vi "_ROSDefinition.vi"() -> ()   [LabVIEW 2013]
uses:
  SubVIs/_ROSDirection.ctl
panel:
  out "Port Count":i32=9
  out "Right Gripper":T1={"Seconds"=1403708875, "NanoSec"=338000000, "ID"=65538, "enabled"=enum."TRUE", "calibrated"=enum."UNKNOWN", "ready"=enum."FALSE", "moving"=enum."TRUE", "gripping"=enum."FALSE", "missed"=enum."UNKNOWN", "error"=enum."FALSE", "reverse"=enum."FALSE", "position"=0.0, "force"=0.0, "state"="{\n  \"error_flags\" : 0,\n  \"op_mode\" : 0\n}", "command"="calibrate", "command sender"="NONA", "command sequence"=3} {"ID" format="%08x"}
  in  "Baxter Topics Old":T3(array[cluster])=[{"Topic"="/robot/head/command_head_nod", "Type"="std_msgs/Bool", "Action"=enum."Publisher"}, {"Topic"="/robot/limb/left/joint_command_mode", "Type"="baxter_msgs/JointCommandMode", "Action"=enum."Publisher"}, {"Topic"="/robot/limb/left/command_joint_angles", "Type"="baxter_msgs/JointPositions", "Action"=enum."Publisher"}, {"Topic"="/robot/limb/right/joint_command_mode", "Type"="baxter_msgs/JointCommandMode", "Action"=enum."Publisher"}, {"Topic"="/robot/limb/right/command_joint_angles", "Type"="baxter_msgs/JointPositions", "Action"=enum."Publisher"}, {"Topic"="/robot/set_super_enable", "Type"="std_msgs/Bool", "Action"=enum."Publisher"}, {"Topic"="/robot/joint_states", "Type"="sensor_msgs/JointState", "Action"=enum."Subscriber"}, {"Topic"="/robot/range/right_hand_range", "Type"="sensor_msgs/Range", "Action"=enum."Subscriber"}, {"Topic"="/robot/range/left_hand_range", "Type"="sensor_msgs/Range", "Action"=enum."Subscriber"}, {"Topic"="/cameras/left_hand_camera/image", "Type"="sensor_msgs/Image", "Action"=enum."Subscriber"}, {"Topic"="/cameras/right_hand_camera/image", "Type"="sensor_msgs/Image", "Action"=enum."Subscriber"}, {"Topic"="/cameras/head_camera/image", "Type"="sensor_msgs/Image", "Action"=enum."Subscriber"}, {"Topic"="/robot/limb/right/accessory/gripper/command_calibrate", "Type"="std_msgs/Bool", "Action"=enum."Publisher"}, {"Topic"="/robot/limb/left/accessory/gripper/command_calibrate", "Type"="std_msgs/Empty", "Action"=enum."Publisher"}, {"Topic"="/robot/limb/left/accessory/gripper/command_goto", "Type"="std_msgs/Float32", "Action"=enum."Publisher"}, {"Topic"="/robot/limb/right/accessory/gripper/command_goto", "Type"="std_msgs/Float32", "Action"=enum."Publisher"}, {"Topic"="/sdk/robot/digital_io/left_lower_cuff/state", "Type"="baxter_msgs/DigitalIOState", "Action"=enum."Subscriber"}, {"Topic"="/sdk/robot/digital_io/right_lower_cuff/state", "Type"="baxter_msgs/DigitalIOState", "Action"=enum."Subscriber"}, {"Topic"="/sdk/robot/digital_io/command", "Type"="baxter_msgs/DigitalOutputCommand", "Action"=enum."Publisher"}, {"Topic"="/sdk/robot/itb/torso_left_itb/state", "Type"="baxter_msgs/ITB", "Action"=enum."Subscriber"}, {"Topic"="/sdk/robot/itb/left_itb/state", "Type"="baxter_msgs/ITB", "Action"=enum."Subscriber"}, {"Topic"="/sdk/robot/itb/torso_right_itb/state", "Type"="baxter_msgs/ITB", "Action"=enum."Subscriber"}, {"Topic"="/sdk/robot/itb/right_itb/state", "Type"="baxter_msgs/ITB", "Action"=enum."Subscriber"}, {"Topic"="/sdk/xdisplay", "Type"="sensor_msgs/Image", "Action"=enum."Publisher"}, {"Topic"="/sdk/robot/digital_io/left_lower_button/state", "Type"="baxter_msgs/DigitalIOState", "Action"=enum."Subscriber"}, {"Topic"="/sdk/robot/digital_io/right_lower_button/state", "Type"="baxter_msgs/DigitalIOState", "Action"=enum."Subscriber"}, {"Topic"="/sdk/robot/digital_io/left_upper_button/state", "Type"="baxter_msgs/DigitalIOState", "Action"=enum."Subscriber"}, {"Topic"="/sdk/robot/digital_io/right_upper_button/state", "Type"="baxter_msgs/DigitalIOState", "Action"=enum."Subscriber"}, {"Topic"="/sdk/robot/limb/right/endpoint/state", "Type"="baxter_msgs/EndpointState", "Action"=enum."Subscriber"}, {"Topic"="/sdk/robot/limb/left/endpoint/state", "Type"="baxter_msgs/EndpointState", "Action"=enum."Subscriber"}, {"Topic"="/sdk/robot/limb/left/accessory/gripper/state", "Type"="baxter_msgs/GripperState", "Action"=enum."Subscriber"}, {"Topic"="/sdk/robot/limb/right/accessory/gripper/state", "Type"="baxter_msgs/GripperState", "Action"=enum."Subscriber"}, {"Topic"="/joint_states", "Type"="sensor_msgs/JointState", "Action"=enum."Subscriber"}, {"Topic"="/sdk/robot/limb/left/solve_ik_position", "Type"="baxter_msgs/SolvePositionIK", "Action"=enum."Service Client"}, {"Topic"="/sdk/robot/limb/right/solve_ik_position", "Type"="baxter_msgs/SolvePositionIK", "Action"=enum."Service Client"}, {"Topic"="/cameras/close", "Type"="baxter_msgs/CloseCamera", "Action"=enum."Service Client"}, {"Topic"="/cameras/open", "Type"="baxter_msgs/OpenCamera", "Action"=enum."Service Client"}, {"Topic"="/cameras/list", "Type"="baxter_msgs/ListCameras", "Action"=enum."Service Client"}, {"Topic"="/robot/sonar/head_sonar/state", "Type"="sensor_msgs/PointCloud", "Action"=enum."Subscriber"}, {"Topic"="/robot/limb/left/command_joint_velocities", "Type"="std_msgs/JointVelocities", "Action"=enum."Publisher"}, {"Topic"="/robot/limb/right/command_joint_velocities", "Type"="std_msgs/JointVelocities", "Action"=enum."Publisher"}, {"Topic"="/robot/sonar/set_lights", "Type"="std_msgs/uint16", "Action"=enum."Publisher"}, {"Topic"="/robot/sonar/set_red_level", "Type"="std_msgs/Float32", "Action"=enum."Publisher"}, {"Topic"="/robot/sonar/set_red_level", "Type"="std_msgs/Float32", "Action"=enum."Publisher"}, {"Topic"="/robot/sonar/set_green_level", "Type"="std_msgs/Float32", "Action"=enum."Publisher"}, {"Topic"="/sdk/robot/head/command_head_pan", "Type"="baxter_msgs/HeadPanCommand", "Action"=enum."Publisher"}, {"Topic"="/sdk/robot/limb/left/accessory/gripper/identity", "Type"="baxter_msgs/GripperIdentity", "Action"=enum."Subscriber"}, {"Topic"="/robot/limb/right/joint_command", "Type"="baxter_msgs/JointCommand", "Action"=enum."Publisher"}, {"Topic"="/robot/limb/left/joint_command", "Type"="baxter_msgs/JointCommand", "Action"=enum."Publisher"}]
  out "Ports":u16[](array[numeric])
  in  "FIFO Size":i32=10
  in  "Active Servers":T4(array[cluster])
  in  "Baxter Topics":T3(array[cluster])=[{"Topic"="/cameras/close", "Type"="baxter_msgs/CloseCamera", "Action"=enum."Service Client"}, {"Topic"="/cameras/head_camera/image", "Type"="sensor_msgs/Image", "Action"=enum."Subscriber"}, {"Topic"="/cameras/left_hand_camera/image", "Type"="sensor_msgs/Image", "Action"=enum."Subscriber"}, {"Topic"="/cameras/list", "Type"="baxter_msgs/ListCameras", "Action"=enum."Service Client"}, {"Topic"="/cameras/open", "Type"="baxter_msgs/OpenCamera", "Action"=enum."Service Client"}, {"Topic"="/cameras/right_hand_camera/image", "Type"="sensor_msgs/Image", "Action"=enum."Subscriber"}, {"Topic"="/joint_states", "Type"="sensor_msgs/JointState", "Action"=enum."Subscriber"}, {"Topic"="/robot/analog_io/left_hand_range/value_uint32", "Type"="std_msgs/Uint32", "Action"=enum."Subscriber"}, {"Topic"="/robot/analog_io/right_hand_range/value_uint32", "Type"="std_msgs/Uint32", "Action"=enum."Subscriber"}, {"Topic"="/robot/digital_io/right_shoulder_button/state", "Type"="baxter_core_msgs/DigitalIOState", "Action"=enum."Subscriber"}, {"Topic"="/robot/end_effector/left_gripper/command", "Type"="baxter_core_msgs/EndEffectorCommand", "Action"=enum."Publisher"}, {"Topic"="/robot/end_effector/right_gripper/command", "Type"="baxter_core_msgs/EndEffectorCommand", "Action"=enum."Publisher"}, {"Topic"="/robot/end_effector/left_gripper/state", "Type"="std_msgs/EndEffectorState", "Action"=enum."Subscriber"}, {"Topic"="/robot/end_effector/right_gripper/state", "Type"="std_msgs/EndEffectorState", "Action"=enum."Subscriber"}, {"Topic"="/robot/head/command_head_nod", "Type"="std_msgs/Bool", "Action"=enum."Publisher"}, {"Topic"="/robot/head/command_head_pan", "Type"="baxter_core_msgs/HeadPanCommand", "Action"=enum."Publisher"}, {"Topic"="/robot/itb/right_itb/state", "Type"="baxter_core_msgs/ITBState", "Action"=enum."Subscriber"}, {"Topic"="/robot/joint_states", "Type"="sensor_msgs/JointState", "Action"=enum."Subscriber"}, {"Topic"="/robot/joint_state_publish_rate", "Type"="std_msgs/Uint16", "Action"=enum."Publisher"}, {"Topic"="/robot/limb/left/accessory/gripper/command_calibrate", "Type"="std_msgs/Empty", "Action"=enum."Publisher"}, {"Topic"="/robot/limb/left/accessory/gripper/command_goto", "Type"="std_msgs/Float32", "Action"=enum."Publisher"}, {"Topic"="/robot/limb/left/joint_command", "Type"="std_msgs/JointCommand", "Action"=enum."Publisher"}, {"Topic"="/robot/limb/right/accessory/gripper/command_calibrate", "Type"="std_msgs/Bool", "Action"=enum."Publisher"}, {"Topic"="/robot/limb/right/accessory/gripper/command_goto", "Type"="std_msgs/Float32", "Action"=enum."Publisher"}, {"Topic"="/robot/limb/right/joint_command", "Type"="baxter_msgs/JointCommand", "Action"=enum."Publisher"}, {"Topic"="/robot/range/left_hand_range", "Type"="sensor_msgs/Range", "Action"=enum."Subscriber"}, {"Topic"="/robot/range/right_hand_range", "Type"="sensor_msgs/Range", "Action"=enum."Subscriber"}, {"Topic"="/robot/set_super_enable", "Type"="std_msgs/Bool", "Action"=enum."Publisher"}, {"Topic"="/robot/sonar/head_sonar/state", "Type"="sensor_msgs/PointCloud", "Action"=enum."Subscriber"}, {"Topic"="/robot/sonar/set_green_level", "Type"="std_msgs/Float32", "Action"=enum."Publisher"}, {"Topic"="/robot/sonar/set_lights", "Type"="std_msgs/uint16", "Action"=enum."Publisher"}, {"Topic"="/robot/sonar/set_red_level", "Type"="std_msgs/Float32", "Action"=enum."Publisher"}, {"Topic"="/robot/sonar/set_red_level", "Type"="std_msgs/Float32", "Action"=enum."Publisher"}, {"Topic"="/sdk/robot/digital_io/command", "Type"="baxter_msgs/DigitalOutputCommand", "Action"=enum."Publisher"}, {"Topic"="/sdk/robot/digital_io/left_lower_button/state", "Type"="baxter_msgs/DigitalIOState", "Action"=enum."Subscriber"}, {"Topic"="/sdk/robot/digital_io/left_lower_cuff/state", "Type"="baxter_msgs/DigitalIOState", "Action"=enum."Subscriber"}, {"Topic"="/sdk/robot/digital_io/left_upper_button/state", "Type"="baxter_msgs/DigitalIOState", "Action"=enum."Subscriber"}, {"Topic"="/sdk/robot/digital_io/right_lower_button/state", "Type"="baxter_msgs/DigitalIOState", "Action"=enum."Subscriber"}, {"Topic"="/sdk/robot/digital_io/right_lower_cuff/state", "Type"="baxter_msgs/DigitalIOState", "Action"=enum."Subscriber"}, {"Topic"="/sdk/robot/digital_io/right_upper_button/state", "Type"="baxter_msgs/DigitalIOState", "Action"=enum."Subscriber"}, {"Topic"="/sdk/robot/head/command_head_pan", "Type"="baxter_msgs/HeadPanCommand", "Action"=enum."Publisher"}, {"Topic"="/sdk/robot/itb/left_itb/state", "Type"="baxter_msgs/ITB", "Action"=enum."Subscriber"}, {"Topic"="/sdk/robot/itb/right_itb/state", "Type"="baxter_msgs/ITB", "Action"=enum."Subscriber"}, {"Topic"="/sdk/robot/itb/torso_left_itb/state", "Type"="baxter_msgs/ITB", "Action"=enum."Subscriber"}, {"Topic"="/sdk/robot/itb/torso_right_itb/state", "Type"="baxter_msgs/ITB", "Action"=enum."Subscriber"}, {"Topic"="/sdk/robot/limb/left/accessory/gripper/identity", "Type"="baxter_msgs/GripperIdentity", "Action"=enum."Subscriber"}, {"Topic"="/sdk/robot/limb/left/accessory/gripper/state", "Type"="baxter_msgs/GripperState", "Action"=enum."Subscriber"}, {"Topic"="/sdk/robot/limb/left/endpoint/state", "Type"="baxter_msgs/EndpointState", "Action"=enum."Subscriber"}, {"Topic"="/sdk/robot/limb/left/solve_ik_position", "Type"="baxter_msgs/SolvePositionIK", "Action"=enum."Service Client"}, {"Topic"="/sdk/robot/limb/right/accessory/gripper/state", "Type"="baxter_msgs/GripperState", "Action"=enum."Subscriber"}, {"Topic"="/sdk/robot/limb/right/endpoint/state", "Type"="baxter_msgs/EndpointState", "Action"=enum."Subscriber"}, {"Topic"="/sdk/robot/limb/right/solve_ik_position", "Type"="baxter_msgs/SolvePositionIK", "Action"=enum."Service Client"}, {"Topic"="/robot/xdisplay", "Type"="sensor_msgs/Image", "Action"=enum."Publisher"}, {"Topic"="/robot/itb/left_itb/state", "Type"="baxter_core_msgs/ITBState", "Action"=enum."Subscriber"}, {"Topic"="", "Type"="", "Action"=enum."Subscriber"}]
  in  "Nodes":cluster{"node":string, "Node Port":u32}[](array[cluster])=[{"node"="/labview", "Node Port"=7000}]
  out "Baxter There?":bool=TRUE
  out "ROS Master":string="192.168.0.12:11311"
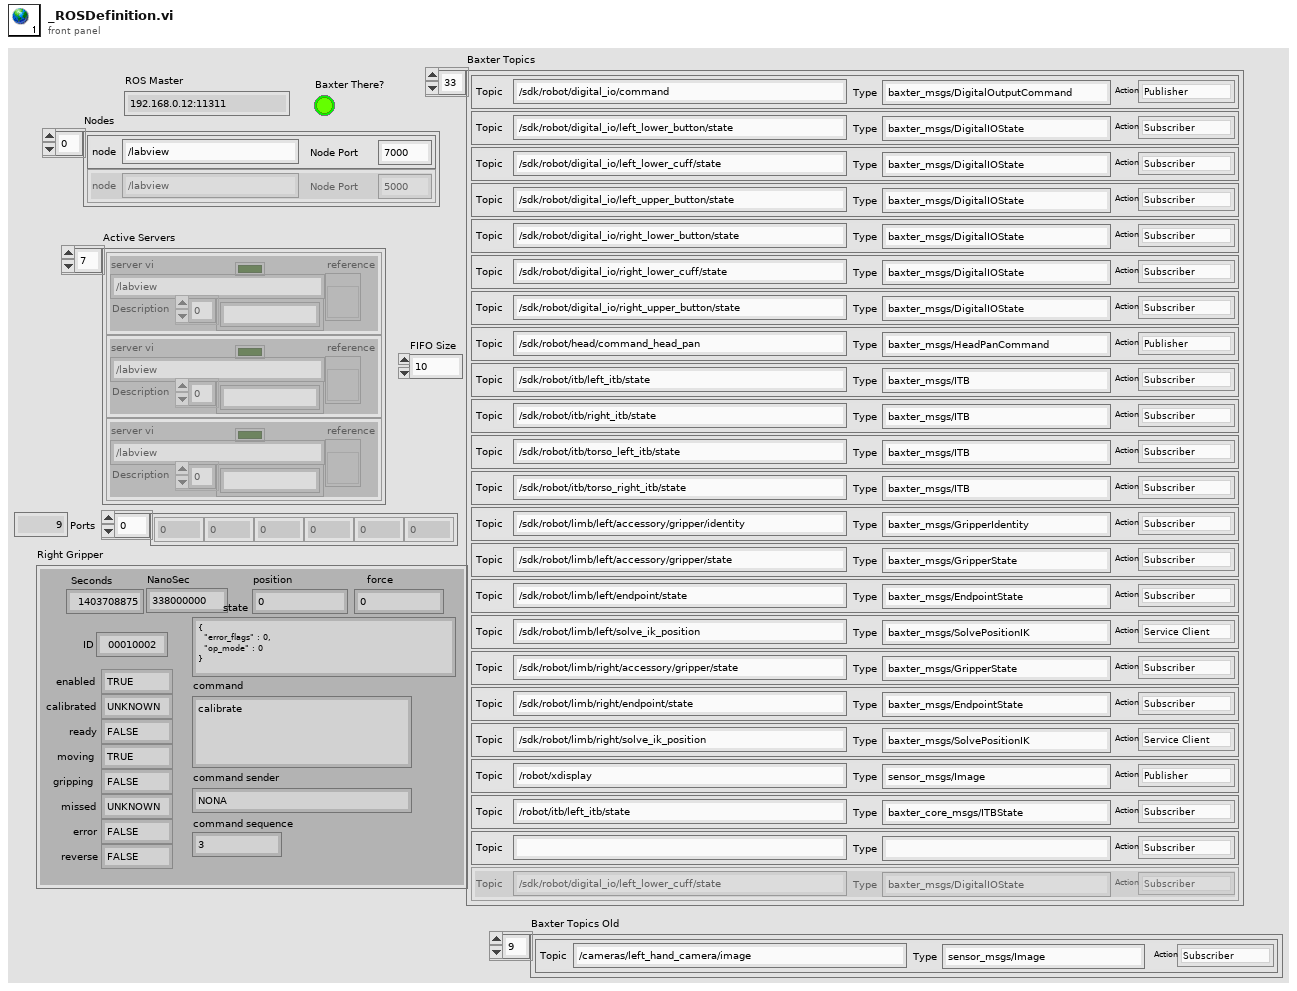
[diagram p1: front panel]
types:
  T1 = cluster{"Seconds":u32, "NanoSec":u32, "ID":u32, "enabled":enum8{"FALSE", "TRUE", "UNKNOWN"}, "calibrated":enum8{"FALSE", "TRUE", "UNKNOWN"}, "ready":enum8{"FALSE", "TRUE", "UNKNOWN"}, "moving":enum8{"FALSE", "TRUE", "UNKNOWN"}, "gripping":enum8{"FALSE", "TRUE", "UNKNOWN"}, "missed":enum8{"FALSE", "TRUE", "UNKNOWN"}, "error":enum8{"FALSE", "TRUE", "UNKNOWN"}, "reverse":enum8{"FALSE", "TRUE", "UNKNOWN"}, "position":sgl, "force":sgl, "state":string, "command":string, "command sender":string, "command sequence":u32}
  T2 = typedef "_ROSDirection.ctl" = enum16{"Node", "Publisher", "Subscriber", "Service Client"}
  T3 = cluster{"Topic":string, "Type":string, "Action":T2}[]
  T4 = cluster{"server vi":string, "reference":refnum<vi>, "Description":string[], "Connected":bool}[]
diagram:
